vi "Control Loop Status Values.vi"(11 "Loop Data in":T1) -> (2 "Status Values":dbl[](array[numeric]), 3 "Loop Data":T1)   [LabVIEW 2020, in "VolatusDaq.lvlib" / "DaqControl.lvclass"]
uses:
  DaqControl.lvclass
  Loop Data.ctl
  Volatus/Event API/EventAPI.lvclass
  Volatus/DataHandlerAPI/DataHandlerAPI.lvclass
  Sequence Action.ctl
  Seq Action Type.ctl
  Value Update.ctl
  Seq Cmd.ctl
  Seq Cmd Type.ctl
  Signal Type.ctl
  DaqControl.lvclass/DaqControl.ctl
  lv-vecto/Vecto/Vecto.lvlib
  VolatusDaq.lvlib
  Sequence.ctl
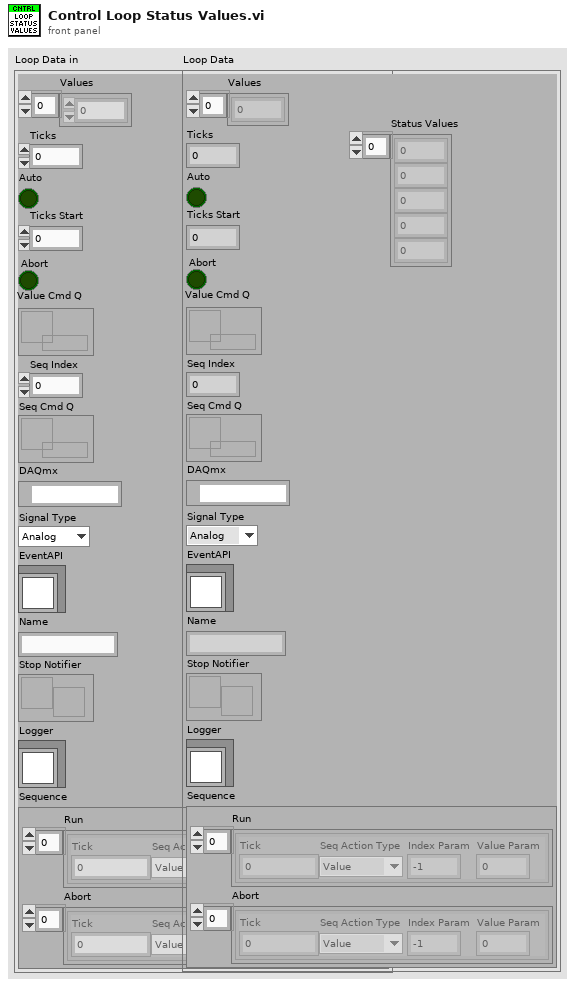
[diagram p1: front panel]
types:
  T1 = typedef "VolatusDaq.lvlib/DaqControl.lvclass/Loop Data.ctl" = cluster{"Values":dbl[], "Ticks":u32, "Auto":bool, "Ticks Start":u32, "Abort":bool, "Value Cmd Q":refnum<queue>, "Seq Index":i32, "Seq Cmd Q":refnum<queue>, "DAQmx":refnum<k21>, "Signal Type":T2, "EventAPI":refnum<class "EventAPI.lvclass">, "Name":string, "Stop Notifier":refnum<notifier>, "Logger":refnum<class "DataHandlerAPI.lvclass">, "Sequence":T3}
  T2 = typedef "VolatusDaq.lvlib/Signal Type.ctl" = enum16{"Analog", "Digital"}
  T3 = typedef "VolatusDaq.lvlib/Sequence.ctl" = cluster{"Run":T4[], "Abort":T4[]}
  T4 = typedef "VolatusDaq.lvlib/Sequence Action.ctl" = cluster{"Tick":u32, "Seq Action Type":T5, "Index Param":i32, "Value Param":dbl}
  T5 = typedef "VolatusDaq.lvlib/Seq Action Type.ctl" = enum16{"Value", "Stop"}
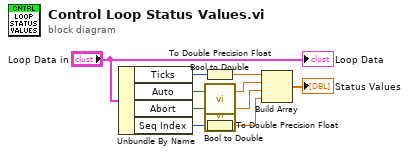
[diagram p0: block diagram]
diagram:
  n1 = Unbundle By Name("Loop Data in") -> ("Ticks"=w7:u32, "Auto"=w9:bool, "Abort"=w8:bool, "Seq Index"=w6:i32)
  n2 = To Double Precision Float(number=w7) -> (double precision float=w5:dbl)
  n3 = call "Bool to Double.vi"("Bool"=w9) -> ("Double"=w4:dbl)  [unwired: 2 in]
  n4 = call "Bool to Double.vi"("Bool"=w8) -> ("Double"=w3:dbl)  [unwired: 2 in]
  n5 = To Double Precision Float(number=w6) -> (double precision float=w2:dbl)
  n6 = Build Array(w5, w4, w3, w2) -> (→"Status Values":dbl[])
  "Loop Data" <- "Loop Data in"
